vi "Option Write Data.vi"(0 "Option Selection":T1, 11 "Error In":errorcluster) -> (8 "appended array":T2[](array[typedef]) {"ERD Number" format="%.0x"}, 15 "Error Out":errorcluster)   [LabVIEW 2016, in "2015 VA Washer.lvlib"]
uses:
  Projects/2015 VA Washer.lvlib
  Common/LabVIEW GEA2 Toolkit/LabVIEW_GEA2_Toolkit.lvlibp/type defs/ERD Write Data In.ctl
  Common/LabVIEW GEA2 Toolkit/LabVIEW_GEA2_Toolkit.lvlibp/type defs/Data Type.ctl
  Controls/Options.ctl
  Common/LabVIEW GEA2 Toolkit/LabVIEW_GEA2_Toolkit.lvlibp
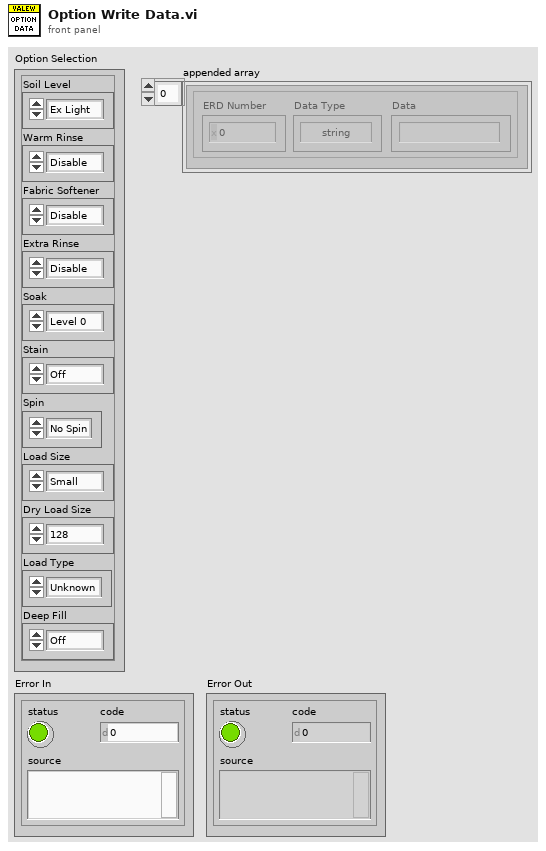
[diagram p1: front panel]
types:
  T1 = typedef "2015 VA Washer.lvlib/Options.ctl" = cluster{"Soil Level":enum8{"Ex Light", "Light", "Normal", "Heavy", "Ex Heavy"}, "Warm Rinse":enum8{"Disable", "Enable"}, "Fabric Softener":enum16{"Disable", "Enable"}, "Extra Rinse":enum8{"Disable", "Enable"}, "Soak":enum8{"Level 0", "Level 1", "Level 2", "Level 3", "Level 4"}, "Stain":enum8{"Off", "Tomato", "Wine", "Blood", "Grass", "Dirt"}, "Spin":enum16{"No Spin", "Normal Spin", "More Spin", "Max Spin"}, "Load Size":enum8{"Small", "Medium", "Large", "Super", "Precise Fill", "Super Plus"}, "Dry Load Size":enum16{"128", "256", "384", "5AA", "6A4", "834", "65535"}, "Load Type":enum8{"Unknown", "Cotton", "Synthetic", "Mixed", "Wet", "Low Flow", "Small", "Medium", "Large", "Super", "Super Plus", "Max"}, "Deep Fill":enum8{"Off", "Incremental Fill", "Max Fill"}}
  T2 = typedef "LabVIEW_GEA2_Toolkit.lvlibp/ERD Write Data In.ctl" = cluster{"ERD Number":u16, "Data Type":T3, "Data":string}
  T3 = typedef "LabVIEW_GEA2_Toolkit.lvlibp/Data Type.ctl" = enum16{"string", "boolean", "uint8_t", "uint16_t", "uint32_t", "uint64_t", "int8_t", "int16_t", "int32_t", "int64_t"}
  T4 = enum8{"Unknown", "Cotton", "Synthetic", "Mixed", "Wet", "Low Flow", "Small", "Medium", "Large", "Super", "Super Plus", "Max"}
  T5 = enum16{"128", "256", "384", "5AA", "6A4", "834", "65535"}
  T6 = enum8{"Small", "Medium", "Large", "Super", "Precise Fill", "Super Plus"}
  T7 = enum8{"Ex Light", "Light", "Normal", "Heavy", "Ex Heavy"}
  T8 = enum8{"Level 0", "Level 1", "Level 2", "Level 3", "Level 4"}
  T9 = enum8{"Off", "Tomato", "Wine", "Blood", "Grass", "Dirt"}
  T10 = enum16{"No Spin", "Normal Spin", "More Spin", "Max Spin"}
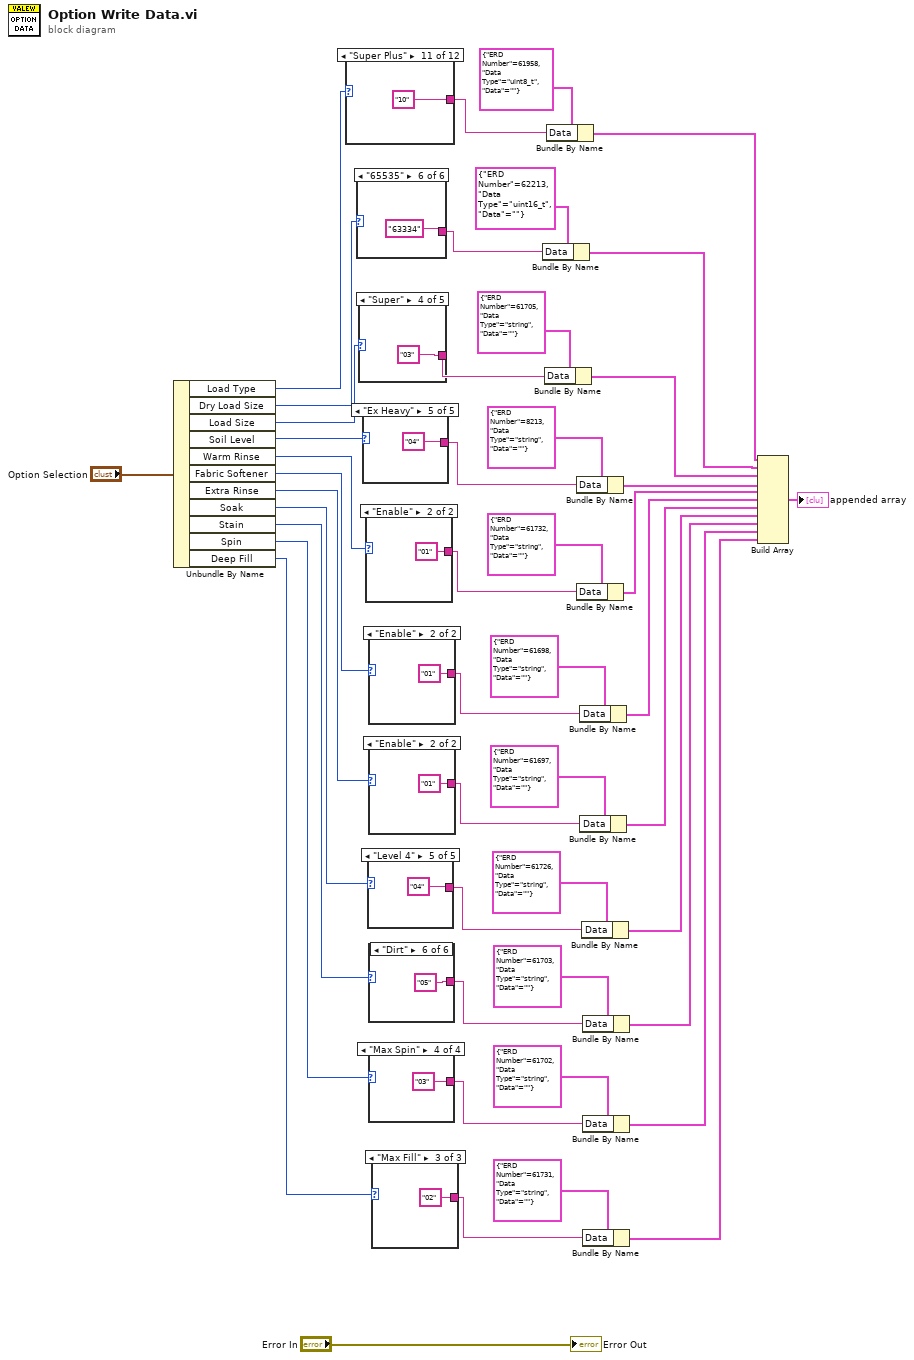
[diagram p0: block diagram]
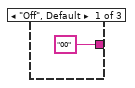
[diagram p2: hidden frame]
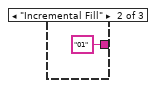
[diagram p3: hidden frame]
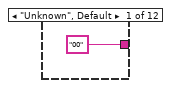
[diagram p4: hidden frame]
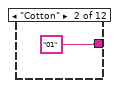
[diagram p5: hidden frame]
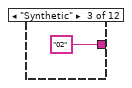
[diagram p6: hidden frame]
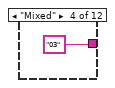
[diagram p7: hidden frame]
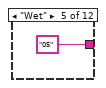
[diagram p8: hidden frame]
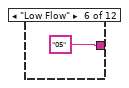
[diagram p9: hidden frame]
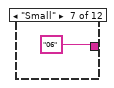
[diagram p10: hidden frame]
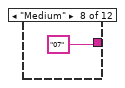
[diagram p11: hidden frame]
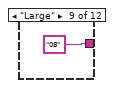
[diagram p12: hidden frame]
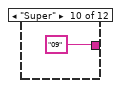
[diagram p13: hidden frame]
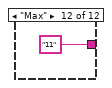
[diagram p14: hidden frame]
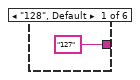
[diagram p15: hidden frame]
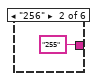
[diagram p16: hidden frame]
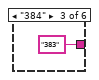
[diagram p17: hidden frame]
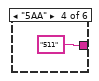
[diagram p18: hidden frame]
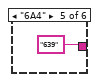
[diagram p19: hidden frame]
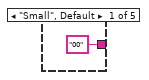
[diagram p20: hidden frame]
diagram:
  n1 = Unbundle By Name("Option Selection") -> ("Load Type"=w10:T4, "Dry Load Size"=w12:T5, "Load Size"=w18:T6, "Soil Level"=w19:T7, "Warm Rinse"=w24:enum8{"Disable", "Enable"}, "Fabric Softener"=w42:enum16{"Disable", "Enable"}, "Extra Rinse"=w43:enum8{"Disable", "Enable"}, "Soak"=w44:T8, "Stain"=w45:T9, "Spin"=w46:T10, "Deep Fill"=w3:enum8{"Off", "Incremental Fill", "Max Fill"})
  n2 = case shown="\"Super Plus\"" w10 {
    tunnel: ["00" "01" "02" "03" "05" "05" "06" "07" "08" "09" "10" "11"] -> w7
    frame "Unknown", Default {
    }
    frame "Cotton" {
    }
    frame "Synthetic" {
    }
    frame "Mixed" {
    }
    frame "Wet" {
    }
    frame "Low Flow" {
    }
    frame "Small" {
    }
    frame "Medium" {
    }
    frame "Large" {
    }
    frame "Super" {
    }
    frame "Super Plus" {
    }
    frame "Max" {
    }
  }
  n3 = case shown="\"65535\"" w12 {
    tunnel: ["127" "255" "383" "511" "639" "63334"] -> w13
    frame "128", Default {
    }
    frame "256" {
    }
    frame "384" {
    }
    frame "5AA" {
    }
    frame "6A4" {
    }
    frame "65535" {
    }
  }
  n4 = case shown="\"Super\"" w18 {
    tunnel: ["00" "01" "02" "03" "04"] -> w16
    frame "Small", Default {
    }
    frame "Medium" {
    }
    frame "Large" {
    }
    frame "Super" {
    }
    frame "Precise Fill" {
    }
  }
  n5 = case shown="\"Ex Heavy\"" w19 {
    tunnel: ["00" "01" "02" "03" "04"] -> w22
    frame "Ex Light", Default {
    }
    frame "Light" {
    }
    frame "Normal" {
    }
    frame "Heavy" {
    }
    frame "Ex Heavy" {
    }
  }
  n6 = case shown="\"Enable\"" w24 {
    tunnel: ["00" "01"] -> w25
    frame "Disable", Default {
    }
    frame "Enable" {
    }
  }
  n7 = case shown="\"Level 4\"" w44 {
    tunnel: ["00" "01" "02" "03" "04"] -> w31
    frame "Level 0", Default {
    }
    frame "Level 1" {
    }
    frame "Level 2" {
    }
    frame "Level 3" {
    }
    frame "Level 4" {
    }
  }
  n8 = case shown="\"Enable\"" w42 {
    tunnel: ["00" "01"] -> w27
    frame "Disable", Default {
    }
    frame "Enable" {
    }
  }
  n9 = case shown="\"Enable\"" w43 {
    tunnel: ["00" "01"] -> w30
    frame "Disable", Default {
    }
    frame "Enable" {
    }
  }
  n10 = case shown="\"Dirt\"" w45 {
    tunnel: ["00" "01" "02" "03" "04" "05"] -> w34
    frame "Off", Default {
    }
    frame "Tomato" {
    }
    frame "Wine" {
    }
    frame "Blood" {
    }
    frame "Grass" {
    }
    frame "Dirt" {
    }
  }
  n11 = case shown="\"Max Spin\"" w46 {
    tunnel: ["00" "01" "02" "03"] -> w35
    frame "No Spin", Default {
    }
    frame "Normal Spin" {
    }
    frame "More Spin" {
    }
    frame "Max Spin" {
    }
  }
  n12 = case shown="\"Max Fill\"" w3 {
    tunnel: ["00" "01" "02"] -> w4
    frame "Off", Default {
    }
    frame "Incremental Fill" {
    }
    frame "Max Fill" {
    }
  }
  n13 = Bundle By Name(cluster=T2 {"ERD Number"=62213, "Data Type"=enum."uint16_t", "Data"=""} ("ERD Write Data In"), "Data"=w13) -> (w11:T2)
  n14 = Bundle By Name(cluster=T2 {"ERD Number"=61705, "Data Type"=enum."string", "Data"=""} ("ERD Write Data In"), "Data"=w16) -> (w15:T2)
  n15 = Bundle By Name(cluster=T2 {"ERD Number"=61958, "Data Type"=enum."uint8_t", "Data"=""} ("ERD Write Data In"), "Data"=w7) -> (w8:T2)
  n16 = Bundle By Name(cluster=T2 {"ERD Number"=8213, "Data Type"=enum."string", "Data"=""} ("ERD Write Data In"), "Data"=w22) -> (w20:T2)
  n17 = Bundle By Name(cluster=T2 {"ERD Number"=61732, "Data Type"=enum."string", "Data"=""} ("ERD Write Data In"), "Data"=w25) -> (w26:T2)
  n18 = Bundle By Name(cluster=T2 {"ERD Number"=61698, "Data Type"=enum."string", "Data"=""} ("ERD Write Data In"), "Data"=w27) -> (w37:T2)
  n19 = Bundle By Name(cluster=T2 {"ERD Number"=61697, "Data Type"=enum."string", "Data"=""} ("ERD Write Data In"), "Data"=w30) -> (w38:T2)
  n20 = Bundle By Name(cluster=T2 {"ERD Number"=61726, "Data Type"=enum."string", "Data"=""} ("ERD Write Data In"), "Data"=w31) -> (w39:T2)
  n21 = Bundle By Name(cluster=T2 {"ERD Number"=61703, "Data Type"=enum."string", "Data"=""} ("ERD Write Data In"), "Data"=w34) -> (w40:T2)
  n22 = Bundle By Name(cluster=T2 {"ERD Number"=61702, "Data Type"=enum."string", "Data"=""} ("ERD Write Data In"), "Data"=w35) -> (w41:T2)
  n23 = Bundle By Name(cluster=T2 {"ERD Number"=61731, "Data Type"=enum."string", "Data"=""} ("ERD Write Data In"), "Data"=w4) -> (w2:T2)
  n24 = Build Array(w8, w11, w15, w20, w26, w37, w38, w39, w40, w41, w2) -> (→"appended array":T2[])
  "Error Out" <- "Error In"
